vi "动力和环境监控系统首页.vi"() -> ()   [LabVIEW 2016, in "环境动力监测库.lvlib"]
uses:
  <vilib>/Utility/miscctls.llb/LVRowAndColumnTypeDef.ctl
  <vilib>/Utility/config.llb/NI_LVConfig.lvlib
  <vilib>/ptbypt/NI_PtbyPt.lvlib
panel:
  out "网络状态":bool
  in  "监测设备更新":bool
  in  "设备列表":i32(listbox)
  in  "add":bool
  out "设备当前时间:":timestamp format="%<%Y/%m/%d %H:%M:%S>T"
  out "当前传感器数量:":i32
  in  "设备":T1(ring)
  # "系统当前状态"
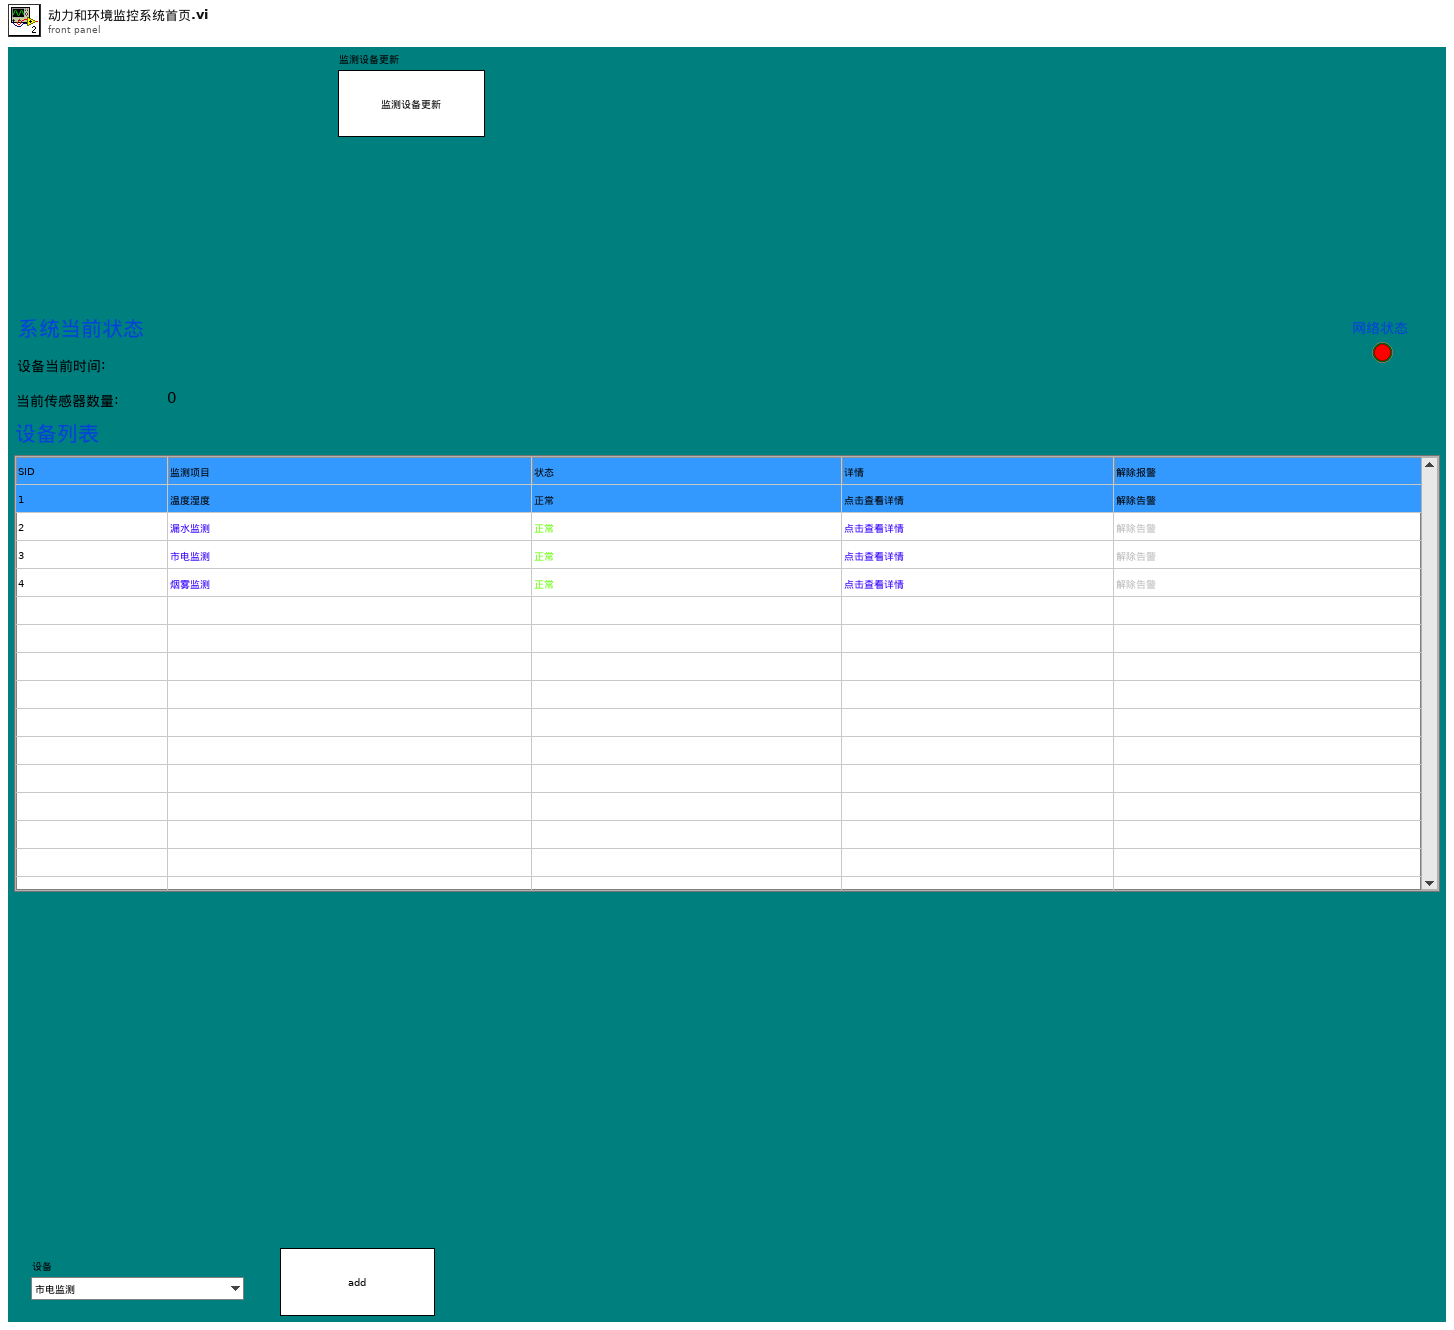
[diagram p1: front panel]
types:
  T1 = enum16{"市电监测", "UPS监测", "用水量监测", "空调监测", "烟雾监测", "温度湿度", "振动监测", "红外入侵监测", "漏水监测", "门禁开关监测", "视频监测"}
  T2 = typedef "NI_LVConfig.lvlib/Config Data RefNum.ctl" = refnum<k1>
  T3 = cluster{"市电监测":bool, "用水量监测":bool, "烟雾监测":bool, "温度湿度":bool, "振动监测":bool, "红外入侵监测":bool, "漏水监测":bool, "门禁开关监测":bool, "视频监测":bool, "UPS监测":bool, "空调监测":bool, "冰箱监测":bool, "排气扇监测":bool, "蓄电池监测":bool}
  T4 = enum32{"Invalid", "Standard", "Closed", "Hidden", "Minimized", "Maximized"}
  T5 = cluster{"漏水监测输出":bool, "门禁监测输出":bool, "温湿度监测输出":bool, "烟雾监测输出":bool, "空调监测输出":bool, "自动重合闸输出":bool, "红外入侵输出":bool, "振动输出":bool}
  T6 = typedef "LVRowAndColumnTypeDef.ctl" = cluster{"Row":i32, "Column":i32}
  T7 = typedef "LVPoint32TypeDef.ctl" = cluster{"Horizontal":i32, "Vertical":i32}
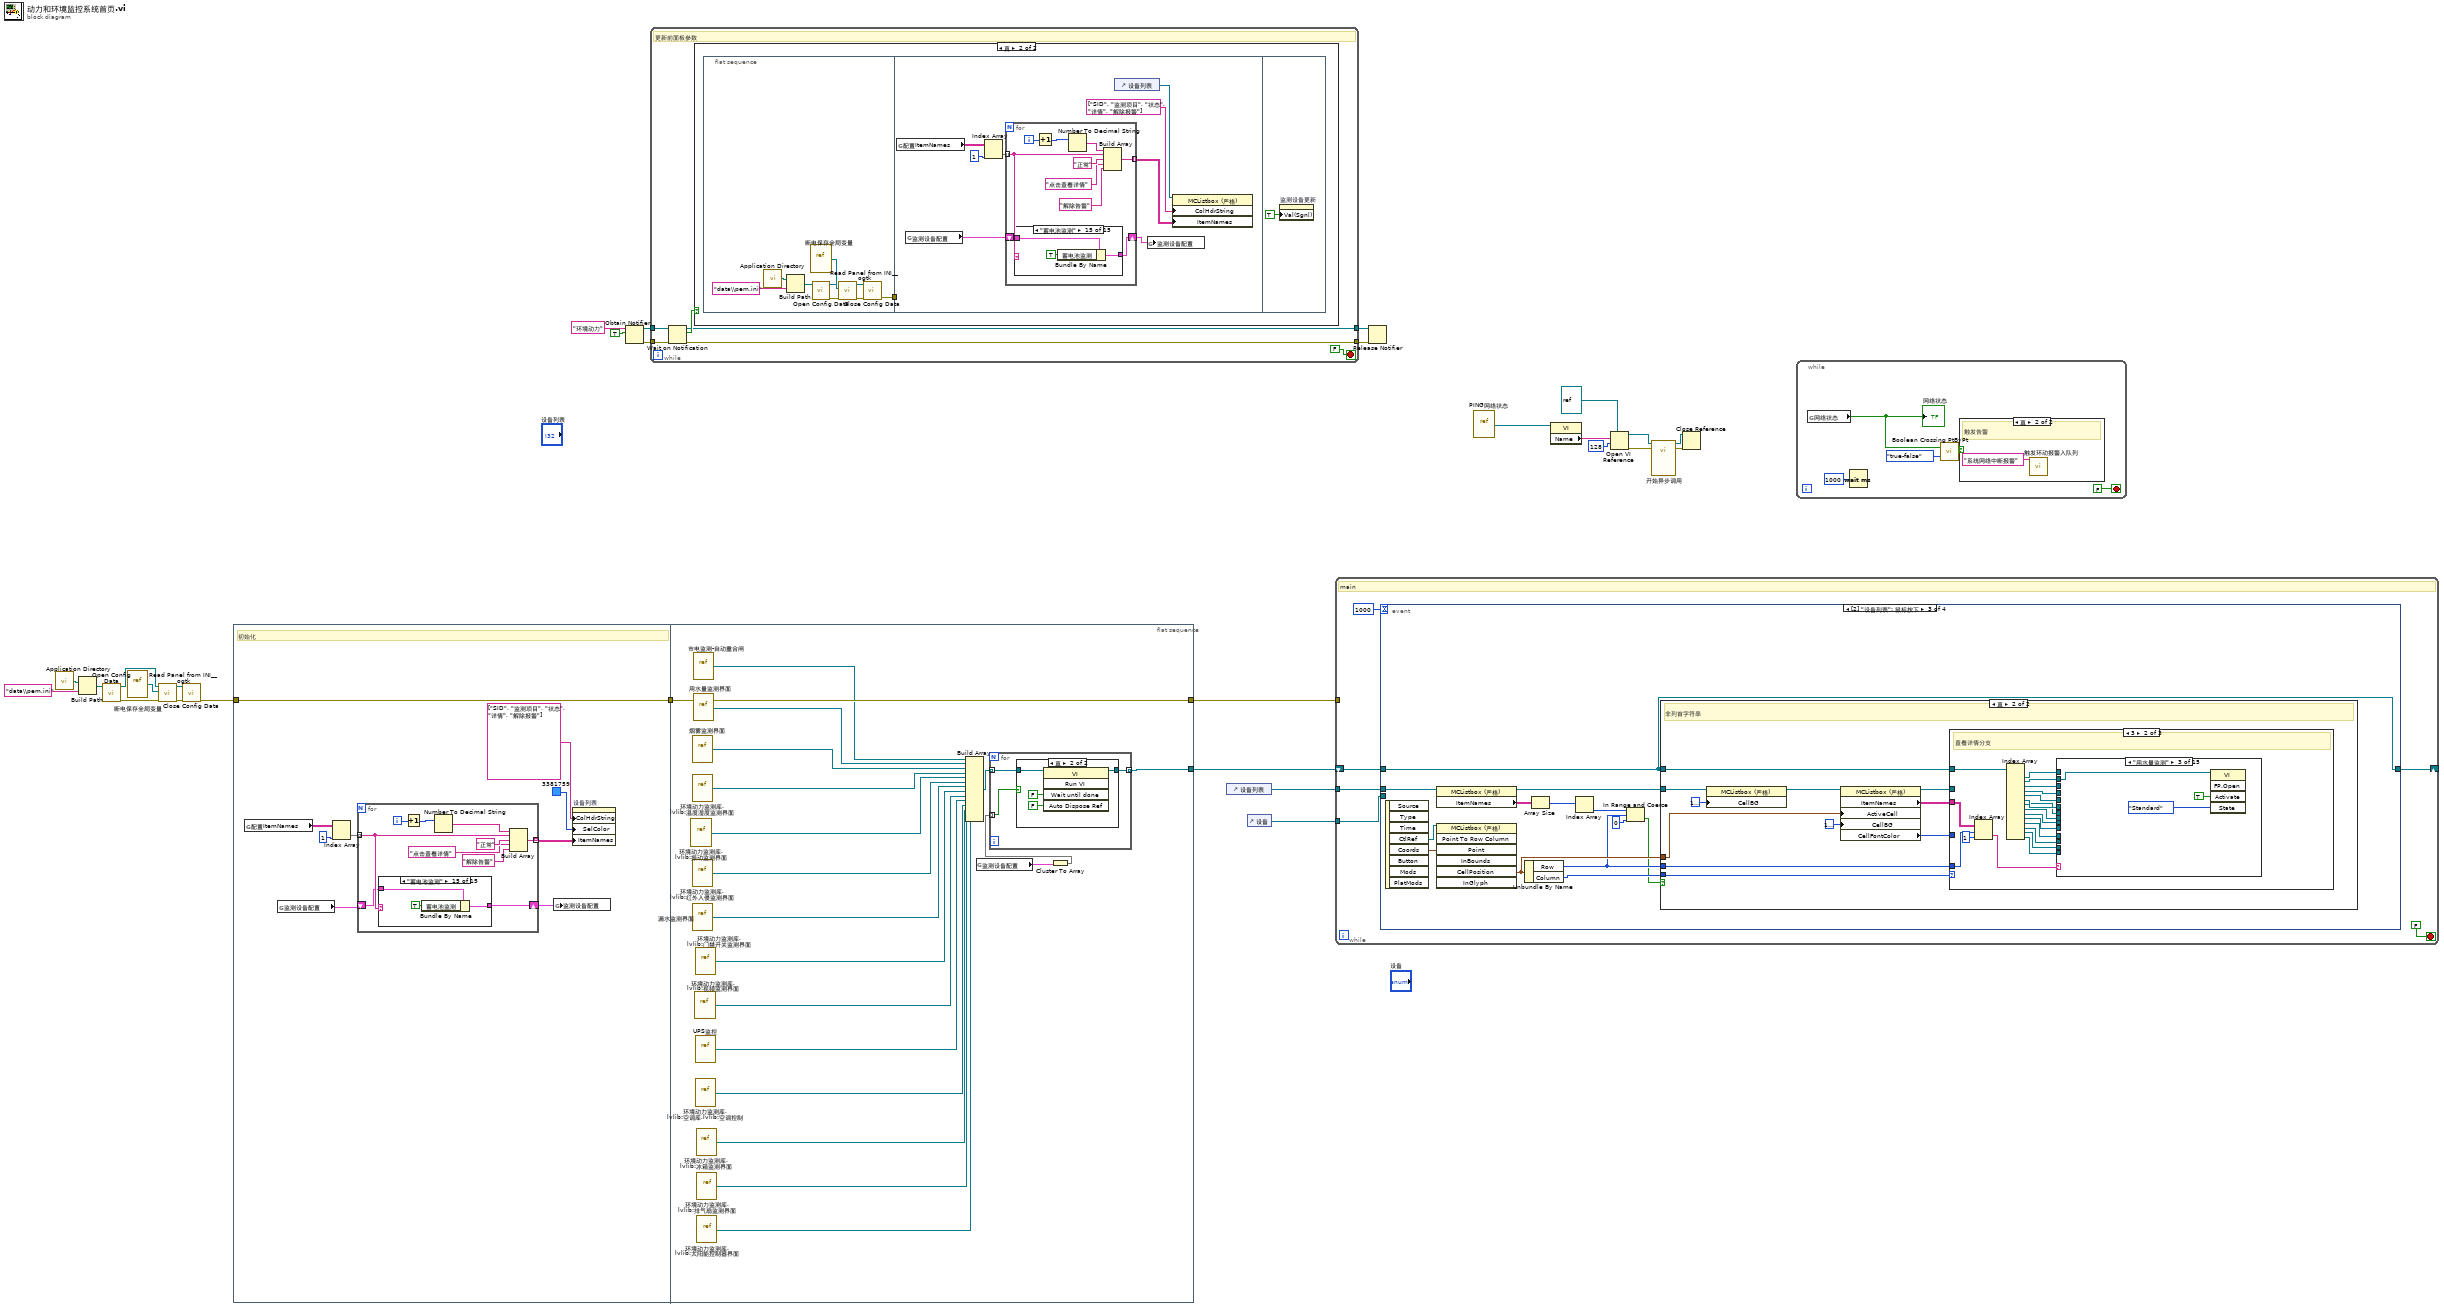
[diagram p0: block diagram]
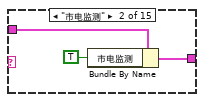
[diagram p5: hidden frame]
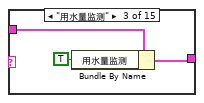
[diagram p6: hidden frame]
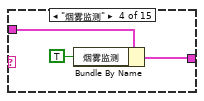
[diagram p7: hidden frame]
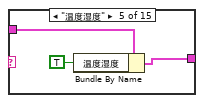
[diagram p8: hidden frame]
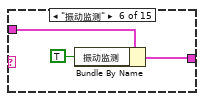
[diagram p9: hidden frame]
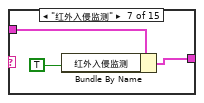
[diagram p10: hidden frame]
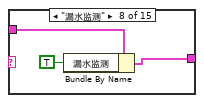
[diagram p11: hidden frame]
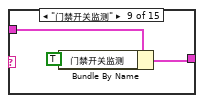
[diagram p12: hidden frame]
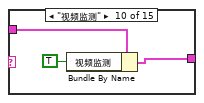
[diagram p13: hidden frame]
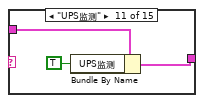
[diagram p14: hidden frame]
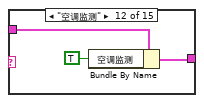
[diagram p15: hidden frame]
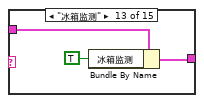
[diagram p16: hidden frame]
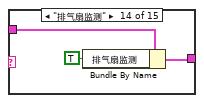
[diagram p17: hidden frame]
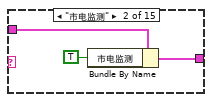
[diagram p19: hidden frame]
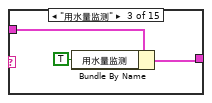
[diagram p20: hidden frame]
diagram:
  n1 = call <vilib>:"Application Directory.vi"() -> ("Application Directory"=w26:path)
  n2 = Build Path(base path=w26, name or relative path="data\\pem.ini" ("名称或相对路径")) -> (appended path=w24:path)
  n3 = call <vilib>:"Open Config Data.vi"("configuration file path"=w24) -> ("error out"=w20:errorcluster, "refnum"=w23:T2)  [unwired: 8 in, 1 out]
  n4 = vi-ref "断电保存全局变量.vi"() -> (w22:refnum<vi>)
  n5 = call <userlib>:"Read Panel from INI__ogtk.vi"("error in (no error)"=w20, "VI ref"=w22, "refnum"=w23) -> ("error out"=w19:errorcluster, "refnum out"=w21:T2)  [unwired: 7 in]
  n6 = call <vilib>:"Close Config Data.vi"("error in (no error)"=w19, "refnum"=w21) -> ("error out"=w18:errorcluster)  [unwired: 8 in, 1 out]
  n7 = flat-sequence {
    tunnel: w18 -> [w31]
    tunnel: [w31] -> w11
    tunnel: [w109] -> w9
    tunnel: w11 -> [w109]
    tunnel: [w95] -> w10
    frame #0 {
      # "初始化"
      n8 = global read "断电保存全局变量.vi" "配置ItemNames"() -> (w35:string[][])
      n9 = global read "断电保存全局变量.vi" "监测设备配置"() -> (w30:T3)
      n10 = Index Array(array=w35, index (col)=1 ("禁用的索引 (列)")) -> (element=w33:string[])  [unwired: 1 in]
      n11 = for {
        tunnel: w33 -> [w40] mode=indexing
        tunnel: [w41] -> w32 mode=indexing
        shift-right: [w38] -> w29
        shift-left: w30 -> [w39]
        i -> [w47]
        n12 = case shown="\"蓄电池监测\"" w40 {
          tunnel: w39 -> [w48 w51 w53 w56 w59 w62 w65 w68 w71 w74 w77 w80 w83 w86 w89]
          tunnel: [w48 w49 w52 w55 w58 w61 w64 w67 w70 w73 w76 w79 w82 w85 w88] -> w38
          frame "假", Default {
          }
          frame "市电监测" {
            n13 = Bundle By Name(cluster=w51, "市电监测"=TRUE) -> (w49:T3)
          }
          frame "用水量监测" {
            n14 = Bundle By Name(cluster=w53, "用水量监测"=TRUE ("市电监测")) -> (w52:T3)
          }
          frame "烟雾监测" {
            n15 = Bundle By Name(cluster=w56, "烟雾监测"=TRUE ("市电监测")) -> (w55:T3)
          }
          frame "温度湿度" {
            n16 = Bundle By Name(cluster=w59, "温度湿度"=TRUE ("市电监测")) -> (w58:T3)
          }
          frame "振动监测" {
            n17 = Bundle By Name(cluster=w62, "振动监测"=TRUE ("市电监测")) -> (w61:T3)
          }
          frame "红外入侵监测" {
            n18 = Bundle By Name(cluster=w65, "红外入侵监测"=TRUE ("市电监测")) -> (w64:T3)
          }
          frame "漏水监测" {
            n19 = Bundle By Name(cluster=w68, "漏水监测"=TRUE ("市电监测")) -> (w67:T3)
          }
          frame "门禁开关监测" {
            n20 = Bundle By Name(cluster=w71, "门禁开关监测"=TRUE ("市电监测")) -> (w70:T3)
          }
          frame "视频监测" {
            n21 = Bundle By Name(cluster=w74, "视频监测"=TRUE ("市电监测")) -> (w73:T3)
          }
          frame "UPS监测" {
            n22 = Bundle By Name(cluster=w77, "UPS监测"=TRUE ("市电监测")) -> (w76:T3)
          }
          frame "空调监测" {
            n23 = Bundle By Name(cluster=w80, "空调监测"=TRUE ("市电监测")) -> (w79:T3)
          }
          frame "冰箱监测" {
            n24 = Bundle By Name(cluster=w83, "冰箱监测"=TRUE ("市电监测")) -> (w82:T3)
          }
          frame "排气扇监测" {
            n25 = Bundle By Name(cluster=w86, "排气扇监测"=TRUE ("市电监测")) -> (w85:T3)
          }
          frame "蓄电池监测" {
            n26 = Bundle By Name(cluster=w89, "蓄电池监测"=TRUE ("市电监测")) -> (w88:T3)
          }
        }
        n27 = Increment(x=w47) -> (x+1=w46:i32)
        n28 = Number To Decimal String(number=w46) -> (decimal integer string=w45:string)  [unwired: 1 in]
        n29 = Build Array(w45, w40, "正常" ("元素"), "点击查看详情" ("元素"), "解除告警" ("元素")) -> (w41:string[])
      }
      n30 = global write "断电保存全局变量.vi" "监测设备配置"(w29) -> ()
      n31 = property on="设备列表" class="MCListbox (严格)"("ColHdrString"=string[] ["SID", "监测项目", "状态", "详情", "解除报警"] ("列首字符串[]"), "SelColor"=u32 3381759, "ItemNames"=w32) -> ()  [unwired: 2 in, 2 out]
    }
    frame #1 {
      n32 = vi-ref "环境动力监测库.lvlib:振动监测界面.vi"() -> (w101:refnum<vi>)
      n33 = vi-ref "烟雾监测界面.vi"() -> (w99:refnum<vi>)
      n34 = vi-ref "环境动力监测库.lvlib:温度湿度监测界面.vi"() -> (w100:refnum<vi>)
      n35 = vi-ref "环境动力监测库.lvlib:红外入侵监测界面.vi"() -> (w102:refnum<vi>)
      n36 = vi-ref "漏水监测界面.vi"() -> (w103:refnum<vi>)
      n37 = vi-ref "市电监测-自动重合闸.vi"() -> (w97:refnum<vi>)
      n38 = vi-ref "用水量监测界面.vi"() -> (w98:refnum<vi>)
      n39 = vi-ref "环境动力监测库.lvlib:视频监测界面.vi"() -> (w105:refnum<vi>)
      n40 = vi-ref "环境动力监测库.lvlib:门禁开关监测界面.vi"() -> (w104:refnum<vi>)
      n41 = vi-ref "UPS监控.vi"() -> (w106:refnum<vi>)
      n42 = vi-ref "环境动力监测库.lvlib:空调库.lvlib:空调控制.vi"() -> (w107:refnum<vi>)
      n43 = vi-ref "环境动力监测库.lvlib:冰箱监测界面.vi"() -> (w92:refnum<vi>)
      n44 = vi-ref "环境动力监测库.lvlib:排气扇监测界面.vi"() -> (w93:refnum<vi>)
      n45 = vi-ref "环境动力监测库.lvlib:太阳能控制器界面.vi"() -> (w94:refnum<vi>)
      n46 = Build Array(w97, w98, w99, w100, w101, w102, w103, w104, w105, w106, w107, w92, w93, w94) -> (w96:refnum<vi>[])
      n47 = global read "断电保存全局变量.vi" "监测设备配置"() -> (w91:T3)
      n48 = Cluster To Array(cluster=w91) -> (array=w108:bool[])
      n49 = for {
        tunnel: w96 -> [w112] mode=indexing
        tunnel: [w111] -> w95 mode=indexing
        tunnel: w108 -> [w110] mode=indexing
        n50 = case shown="真" w110 {
          tunnel: w112 -> [w113 w115]
          tunnel: [w113 w114] -> w111
          frame False {
          }
          frame True {
            n51 = invoke class="VI" method="Run VI"(reference=w115, "Wait until done"=FALSE ("结束前等待"), "Auto Dispose Ref"=FALSE ("自动销毁引用")) -> (reference out=w114:refnum<vi>)  [unwired: 2 in, 4 out]
          }
        }
      }
    }
  }
  n52 = Obtain Notifier(name (unnamed)="环境动力" ("名称（未命名）"), notification data type=TRUE) -> (notifier out=w17:refnum<notifier>, error out=w16:errorcluster)  [unwired: 2 in, 1 out]
  n53 = while {
    tunnel: w17 -> [w123]
    tunnel: w16 -> [w122]
    tunnel: [w119] -> w13
    tunnel: [w118] -> w12
    stop <- FALSE stop-if-true
    # "更新前面板参数"
    n54 = Wait on Notification(notifier=w123, error in (no error)=w122) -> (notifier out=w119:refnum<notifier>, notification=w121:bool, error out=w118:errorcluster)  [unwired: 2 in, 1 out]
    n55 = case shown="真" w121 {
      frame False {
      }
      frame True {
        n56 = flat-sequence {
          tunnel: [w125] -> w124
          tunnel: w124 -> [_]
          frame #0 {
            n57 = call <vilib>:"Application Directory.vi"() -> ("Application Directory"=w126:path)
            n58 = Build Path(base path=w126, name or relative path="data\\pem.ini" ("名称或相对路径")) -> (appended path=w128:path)
            n59 = vi-ref "断电保存全局变量.vi"() -> (w130:refnum<vi>)
            n60 = call <vilib>:"Open Config Data.vi"("configuration file path"=w128) -> ("error out"=w132:errorcluster, "refnum"=w129:T2)  [unwired: 8 in, 1 out]
            n61 = call <userlib>:"Read Panel from INI__ogtk.vi"("error in (no error)"=w132, "VI ref"=w130, "refnum"=w129) -> ("error out"=w133:errorcluster, "refnum out"=w131:T2)  [unwired: 7 in]
            n62 = call <vilib>:"Close Config Data.vi"("error in (no error)"=w133, "refnum"=w131) -> ("error out"=w125:errorcluster)  [unwired: 8 in, 1 out]
          }
          frame #1 {
            n63 = global read "断电保存全局变量.vi" "配置ItemNames"() -> (w136:string[][])
            n64 = global read "断电保存全局变量.vi" "监测设备配置"() -> (w135:T3)
            n65 = Index Array(array=w136, index (col)=1 ("禁用的索引 (列)")) -> (element=w138:string[])  [unwired: 1 in]
            n66 = for {
              tunnel: w138 -> [w142] mode=indexing
              tunnel: [w145] -> w141 mode=indexing
              shift-right: [w143] -> w134
              shift-left: w135 -> [w144]
              i -> [w151]
              n67 = case shown="\"蓄电池监测\"" w142 {
                tunnel: w144 -> [w152 w155 w157 w160 w163 w166 w169 w172 w175 w178 w181 w184 w187 w190 w193]
                tunnel: [w152 w153 w156 w159 w162 w165 w168 w171 w174 w177 w180 w183 w186 w189 w192] -> w143
                frame "假", Default {
                }
                frame "市电监测" {
                  n68 = Bundle By Name(cluster=w155, "市电监测"=TRUE) -> (w153:T3)
                }
                frame "用水量监测" {
                  n69 = Bundle By Name(cluster=w157, "用水量监测"=TRUE ("市电监测")) -> (w156:T3)
                }
                frame "烟雾监测" {
                  n70 = Bundle By Name(cluster=w160, "烟雾监测"=TRUE ("市电监测")) -> (w159:T3)
                }
                frame "温度湿度" {
                  n71 = Bundle By Name(cluster=w163, "温度湿度"=TRUE ("市电监测")) -> (w162:T3)
                }
                frame "振动监测" {
                  n72 = Bundle By Name(cluster=w166, "振动监测"=TRUE ("市电监测")) -> (w165:T3)
                }
                frame "红外入侵监测" {
                  n73 = Bundle By Name(cluster=w169, "红外入侵监测"=TRUE ("市电监测")) -> (w168:T3)
                }
                frame "漏水监测" {
                  n74 = Bundle By Name(cluster=w172, "漏水监测"=TRUE ("市电监测")) -> (w171:T3)
                }
                frame "门禁开关监测" {
                  n75 = Bundle By Name(cluster=w175, "门禁开关监测"=TRUE ("市电监测")) -> (w174:T3)
                }
                frame "视频监测" {
                  n76 = Bundle By Name(cluster=w178, "视频监测"=TRUE ("市电监测")) -> (w177:T3)
                }
                frame "UPS监测" {
                  n77 = Bundle By Name(cluster=w181, "UPS监测"=TRUE ("市电监测")) -> (w180:T3)
                }
                frame "空调监测" {
                  n78 = Bundle By Name(cluster=w184, "空调监测"=TRUE ("市电监测")) -> (w183:T3)
                }
                frame "冰箱监测" {
                  n79 = Bundle By Name(cluster=w187, "冰箱监测"=TRUE ("市电监测")) -> (w186:T3)
                }
                frame "排气扇监测" {
                  n80 = Bundle By Name(cluster=w190, "排气扇监测"=TRUE ("市电监测")) -> (w189:T3)
                }
                frame "蓄电池监测" {
                  n81 = Bundle By Name(cluster=w193, "蓄电池监测"=TRUE ("市电监测")) -> (w192:T3)
                }
              }
              n82 = Increment(x=w151) -> (x+1=w150:i32)
              n83 = Number To Decimal String(number=w150) -> (decimal integer string=w149:string)  [unwired: 1 in]
              n84 = Build Array(w149, w142, "正常" ("元素"), "点击查看详情" ("元素"), "解除告警" ("元素")) -> (w145:string[])
            }
            n85 = control-ref of="设备列表"() -> (w139:refnum<vi>)
            n86 = global write "断电保存全局变量.vi" "监测设备配置"(w134) -> ()
            n87 = property class="MCListbox (严格)"(reference=w139, "ColHdrString"=string[] ["SID", "监测项目", "状态", "详情", "解除报警"] ("列首字符串[]"), "ItemNames"=w141) -> ()  [unwired: 1 in, 2 out]
          }
          frame #2 {
            n88 = property on="监测设备更新" class="Bool (严格)"("Val(Sgnl)"=TRUE ("值(信号)")) -> ()  [unwired: 2 in, 2 out]
          }
        }
      }
    }
  }
  n89 = control-ref of="设备列表"() -> (w28:refnum<vi>)
  n90 = control-ref of="设备"() -> (w27:refnum<vi>)
  n91 = while {
    tunnel: w28 -> [w200]
    tunnel: w27 -> [w199]
    tunnel: w9 -> [_]
    shift-right: [w196] -> _
    shift-left: w10 -> [w197]
    stop <- FALSE stop-if-true
    # "main"
    n92 = event shown="[2] \"设备列表\": 鼠标按下" {
      selector: _ -> [_ _ _ _]
      dyn-events: _ -> [_ _ _ _]
      timeout: 1000 -> [_ _ _ _]
      tunnel: w200 -> [_ w284 w291 _]
      tunnel: w199 -> [_ w283 _ _]
      tunnel: w197 -> [w203 w258 w285 w388]
      tunnel: [w203 w258 w285 w387] -> w196
      event Timeout {
        n93 = event-data() -> ()  [unwired: 1 in, 3 out]
        n94 = Get Date/Time In Seconds() -> (seconds since 1Jan1904=→"设备当前时间:":timestamp)
        n95 = property on="设备列表" class="MCListbox (严格)"() -> (error out=w205:errorcluster, "ItemNames"=w214:string[][])  [unwired: 2 in, 1 out]
        n96 = global read "断电保存全局变量.vi" "监测配置输出"() -> (w202:T5)
        n97 = Array Size(array=w214) -> (size(s)=w220:i32[])
        n98 = Index Array(array=w214, index (col) #1=1 ("禁用的索引 (列)"), index (col) #2=2 ("索引 (列)")) -> (element #1=w212:string[], element #2=w210:string[])  [unwired: 2 in]
        n99 = Index Array(array=w220) -> (element=w215:i32)  [unwired: 1 in]
        "当前传感器数量:" <- w215
        n100 = for {
          tunnel: w212 -> [w236] mode=indexing
          tunnel: w202 -> [w235]
          shift-right: [w231] -> w207
          shift-left: w210 -> [w233]
          tunnel: w205 -> [w227]
          tunnel: [w226] -> w204
          i -> [w224]
          w225 = T6 {"Row"=0, "Column"=0} ("活动单元格:活动单元格")
          n101 = case shown="\"烟雾监测\"" w236 {
            tunnel: w235 -> [_ w245 w247 w249 w251 w253 w255]
            tunnel: [TRUE ("烟雾监测输出") w244 w246 w248 w250 w252 w254] -> w234
            frame "假", Default {
            }
            frame "市电监测" {
              n102 = Unbundle By Name(w245) -> ("自动重合闸输出"=w244:bool)
            }
            frame "空调监测" {
              n103 = Unbundle By Name(w247) -> ("空调监测输出"=w246:bool)
            }
            frame "漏水监测" {
              n104 = Unbundle By Name(w249) -> ("漏水监测输出"=w248:bool)
            }
            frame "门禁开关监测" {
              n105 = Unbundle By Name(w251) -> ("门禁监测输出"=w250:bool)
            }
            frame "温度湿度" {
              n106 = Unbundle By Name(w253) -> ("温湿度监测输出"=w252:bool)
            }
            frame "烟雾监测" {
              n107 = Unbundle By Name(w255) -> ("烟雾监测输出"=w254:bool)
            }
          }
          n108 = case shown="假" w234 {
            tunnel: ["报警" "正常"] -> w232
            tunnel: [u32 16711680 u32 6618880] -> w228
            tunnel: [u32 3342591 ("颜色盒") u32 12369084] -> w221
            frame False {
            }
            frame True {
            }
          }
          n109 = Bundle By Name(cluster=w225, "Row"=w224, "Column"=2) -> (w229:T6)
          n110 = Bundle By Name(cluster=w225, "Row"=w224, "Column"=4) -> (w222:T6)
          n111 = property on="设备列表" class="MCListbox (严格)"(error in=w227, "ActiveCell"=w229, "CellFontColor"=w228, "ActiveCell"=w222, "CellFontColor"=w221) -> (error out=w226:errorcluster)  [unwired: 1 in, 1 out]
          n112 = Replace Array Subset(array=w233, new element=w232, index=w224) -> (w231:string[])
        }
        n113 = for {
          N: w215 -> [_]
          tunnel: [w256] -> w219 mode=indexing
          i -> [w257]
          n114 = Increment(x=w257) -> (x+1=w256:i32)
        }
        n115 = Number To Decimal String(number=w219) -> (decimal integer string=w218:string[])  [unwired: 1 in]
        n116 = Replace Array Subset(array=w214, new element=w218, index (col)=0 ("禁用的索引 (列)")) -> (w209:string[][])  [unwired: 1 in]
        n117 = Replace Array Subset(array=w209, new element=w207, index (col)=2 ("禁用的索引 (列)")) -> (w206:string[][])  [unwired: 1 in]
        n118 = property on="设备列表" class="MCListbox (严格)"(error in=w204, "ItemNames"=w206) -> ()  [unwired: 1 in, 2 out]
      }
      event "add": Value Change {
        w260 = u32 3342591 ("颜色盒")
        n119 = event-data() -> ()  [unwired: 1 in, 6 out]
        n120 = property class="MCListbox (严格)"(reference=w284) -> (reference out=w273:refnum<vi>, "ItemNames"=w277:string[][])  [unwired: 1 in, 1 out]
        n121 = property class="Enum (严格)"(reference=w283) -> ("RingText.Text"=w282:string)  [unwired: 1 in, 2 out]
        n122 = Array Size(array=w277) -> (size(s)=w276:i32[])
        n123 = Index Array(array=w276) -> (element=w265:i32)  [unwired: 1 in]
        n124 = Increment(x=w265) -> (x+1=w275:i32)
        n125 = Number To Decimal String(number=w275) -> (decimal integer string=w274:string)  [unwired: 1 in]
        n126 = Build Array(w274, w282, "正常" ("元素"), "点击查看详情" ("元素"), "解除告警" ("元素")) -> (w281:string[])
        n127 = Build Array (concatenate)(w277, w281) -> (w262:string[][])
        n128 = Bundle(w265, "Column"=1) -> (w261:cluster{i32, "Column":i32})  [unwired: 1 in]
        n129 = Bundle(w265, "Column"=2) -> (w270:cluster{i32, "Column":i32})  [unwired: 1 in]
        n130 = Bundle(w265, "Column"=3) -> (w267:cluster{i32, "Column":i32})  [unwired: 1 in]
        n131 = Bundle(w265, "Column"=4) -> (w264:cluster{i32, "Column":i32})  [unwired: 1 in]
        n132 = property class="MCListbox (严格)"(reference=w273, "ItemNames"=w262, "ActiveCell"=w261, "CellFontColor"=w260, "CellFontBold"=TRUE ("活动单元格:单元格字体:斜体"), "ActiveCell"=w270, "CellFontColor"=u32 61277 ("颜色盒"), "ActiveCell"=w267, "CellFontColor"=w260, "ActiveCell"=w264, "CellFontColor"=u32 12369084 ("颜色盒")) -> ()  [unwired: 1 in, 2 out]
      }
      event "设备列表": Mouse Down {
        n133 = event-data() -> ("CtlRef"=w297:refnum<vi>, "Coords"=w295:T7)  [unwired: 1 in, 6 out]
        n134 = property class="MCListbox (严格)"(reference=w291) -> (reference out=w287:refnum<vi>, "ItemNames"=w290:string[][])  [unwired: 1 in, 1 out]
        n135 = invoke class="MCListbox (严格)" method="Point To Row Column"(reference=w297, "Point"=w295) -> ("CellPosition"=w294:T6)  [unwired: 5 in, 6 out]
        n136 = Unbundle By Name(w294) -> ("Row"=w293:i32, "Column"=w296:i32)
        n137 = Array Size(array=w290) -> (size(s)=w289:i32[])
        n138 = Index Array(array=w289) -> (element=w288:i32)  [unwired: 1 in]
        n139 = In Range and Coerce(upper limit=w288, x=w293, lower limit=0 ("下限")) -> (In Range?=w286:bool)  [unwired: 1 out]
        n140 = case shown="真" w286 {
          tunnel: w296 -> [_ w307]
          tunnel: w293 -> [_ w306]
          tunnel: w294 -> [_ w304]
          tunnel: w287 -> [_ w301]
          tunnel: w285 -> [_ w298]
          frame False {
          }
          frame True {
            # "非列首字符串"
            n141 = property class="MCListbox (严格)"(reference=w301, "CellBG"=u32 16777216) -> (reference out=w302:refnum<vi>)  [unwired: 1 in, 1 out]
            n142 = property class="MCListbox (严格)"(reference=w302, "ActiveCell"=w304, "CellBG"=u32 16777216) -> (reference out=w305:refnum<vi>, "ItemNames"=w308:string[][], "CellFontColor"=w299:u32)  [unwired: 1 in, 1 out]
            n143 = case shown="3" w307 {
              tunnel: w308 -> [_ w327 w378]
              tunnel: w306 -> [_ w325 w376]
              tunnel: w305 -> [_ _ w377]
              tunnel: w299 -> [_ _ w375]
              tunnel: w298 -> [_ w323 _]
              frame 0, Default {
              }
              frame 3 {
                # "查看详情分支"
                n144 = Index Array(array=w327, index (row)=w325, index (col)=1 ("禁用的索引 (列)")) -> (element=w324:string)
                n145 = Index Array(array=w323) -> (element #1=w322:refnum<vi>, element #2=w321:refnum<vi>, element #3=w320:refnum<vi>, element #4=w319:refnum<vi>, element #5=w318:refnum<vi>, element #6=w317:refnum<vi>, element #7=w316:refnum<vi>, element #8=w315:refnum<vi>, element #9=w314:refnum<vi>, element #10=w313:refnum<vi>, element #11=w312:refnum<vi>, element #12=w311:refnum<vi>, element #13=w309:refnum<vi>, element #14=w310:refnum<vi>)  [unwired: 14 in]
                n146 = case shown="\"用水量监测\"" w324 {
                  selector: w324 -> [w328 _ _ _ _ _ _ _ _ _ _ _ _ _ _]
                  tunnel: w322 -> [_ w331 _ _ _ _ _ _ _ _ _ _ _ _ _]
                  tunnel: w321 -> [_ _ w334 _ _ _ _ _ _ _ _ _ _ _ _]
                  tunnel: w320 -> [_ _ _ w337 _ _ _ _ _ _ _ _ _ _ _]
                  tunnel: w319 -> [_ _ _ _ w340 _ _ _ _ _ _ _ _ _ _]
                  tunnel: w318 -> [_ _ _ _ _ w343 _ _ _ _ _ _ _ _ _]
                  tunnel: w317 -> [_ _ _ _ _ _ w346 _ _ _ _ _ _ _ _]
                  tunnel: w316 -> [_ _ _ _ _ _ _ w349 _ _ _ _ _ _ _]
                  tunnel: w315 -> [_ _ _ _ _ _ _ _ w352 _ _ _ _ _ _]
                  tunnel: w314 -> [_ _ _ _ _ _ _ _ _ w355 _ _ _ _ _]
                  tunnel: w313 -> [_ _ _ _ _ _ _ _ _ _ w358 _ _ _ _]
                  tunnel: w312 -> [_ _ _ _ _ _ _ _ _ _ _ w361 _ _ _]
                  tunnel: w311 -> [_ _ _ _ _ _ _ _ _ _ _ _ w364 _ _]
                  tunnel: w310 -> [_ _ _ _ _ _ _ _ _ _ _ _ _ _ w370]
                  tunnel: w309 -> [_ _ _ _ _ _ _ _ _ _ _ _ _ w367 _]
                  frame "假", Default {
                    n147 = Concatenate Strings(w328, "详情" ("字符串")) -> (w330:string)
                    n148 = One Button Dialog(message=w330) -> ()  [unwired: 1 in, 1 out]
                  }
                  frame "市电监测" {
                    n149 = invoke class="VI" method="FP.Open"(reference=w331, "Activate"=TRUE ("激活？"), "State"=T4."Standard" ("状态")) -> ()  [unwired: 2 in, 5 out]
                  }
                  frame "用水量监测" {
                    n150 = invoke class="VI" method="FP.Open"(reference=w334, "Activate"=TRUE ("激活？"), "State"=T4."Standard" ("状态")) -> ()  [unwired: 2 in, 5 out]
                  }
                  frame "烟雾监测" {
                    n151 = invoke class="VI" method="FP.Open"(reference=w337, "Activate"=TRUE ("激活？"), "State"=T4."Standard" ("状态")) -> ()  [unwired: 2 in, 5 out]
                  }
                  frame "温度湿度" {
                    n152 = invoke class="VI" method="FP.Open"(reference=w340, "Activate"=TRUE ("激活？"), "State"=T4."Standard" ("状态")) -> ()  [unwired: 2 in, 5 out]
                  }
                  frame "振动监测" {
                    n153 = invoke class="VI" method="FP.Open"(reference=w343, "Activate"=TRUE ("激活？"), "State"=T4."Standard" ("状态")) -> ()  [unwired: 2 in, 5 out]
                  }
                  frame "红外入侵监测" {
                    n154 = invoke class="VI" method="FP.Open"(reference=w346, "Activate"=TRUE ("激活？"), "State"=T4."Standard" ("状态")) -> ()  [unwired: 2 in, 5 out]
                  }
                  frame "漏水监测" {
                    n155 = invoke class="VI" method="FP.Open"(reference=w349, "Activate"=TRUE ("激活？"), "State"=T4."Standard" ("状态")) -> ()  [unwired: 2 in, 5 out]
                  }
                  frame "门禁开关监测" {
                    n156 = invoke class="VI" method="FP.Open"(reference=w352, "Activate"=TRUE ("激活？"), "State"=T4."Standard" ("状态")) -> ()  [unwired: 2 in, 5 out]
                  }
                  frame "视频监测" {
                    n157 = invoke class="VI" method="FP.Open"(reference=w355, "Activate"=TRUE ("激活？"), "State"=T4."Standard" ("状态")) -> ()  [unwired: 2 in, 5 out]
                  }
                  frame "UPS监测" {
                    n158 = invoke class="VI" method="FP.Open"(reference=w358, "Activate"=TRUE ("激活？"), "State"=T4."Standard" ("状态")) -> ()  [unwired: 2 in, 5 out]
                  }
                  frame "空调监测" {
                    n159 = invoke class="VI" method="FP.Open"(reference=w361, "Activate"=TRUE ("激活？"), "State"=T4."Standard" ("状态")) -> ()  [unwired: 2 in, 5 out]
                  }
                  frame "冰箱监测" {
                    n160 = invoke class="VI" method="FP.Open"(reference=w364, "Activate"=TRUE ("激活？"), "State"=T4."Standard" ("状态")) -> ()  [unwired: 2 in, 5 out]
                  }
                  frame "排气扇监测" {
                    n161 = invoke class="VI" method="FP.Open"(reference=w367, "Activate"=TRUE ("激活？"), "State"=T4."Standard" ("状态")) -> ()  [unwired: 2 in, 5 out]
                  }
                  frame "蓄电池监测" {
                    n162 = invoke class="VI" method="FP.Open"(reference=w370, "Activate"=TRUE ("激活？"), "State"=T4."Standard" ("状态")) -> ()  [unwired: 2 in, 5 out]
                  }
                }
              }
              frame 4 {
                # "解除报警"
                n163 = Equal?(x=w375, y=u32 3342591 ("颜色盒")) -> (x = y?=w374:bool)
                n164 = case shown="真" w374 {
                  tunnel: w378 -> [_ w383]
                  tunnel: w377 -> [_ _]
                  tunnel: w376 -> [_ w382]
                  frame False {
                  }
                  frame True {
                    n165 = Index Array(array=w383, index (row)=w382, index (col)=1 ("禁用的索引 (列)")) -> (element=w380:string)
                    n166 = Format Into String(format string="是否解除%s报警？" ("消息"), w380) -> (resulting string=w384:string)  [unwired: 2 in, 1 out]
                    n167 = Two Button Dialog(message=w384) -> (T button?=w379:bool)  [unwired: 2 in]
                    n168 = case shown="真" w379 {
                      frame False {
                      }
                      frame True {
                        # "触发解除报警事件"
                      }
                    }
                  }
                }
              }
            }
          }
        }
      }
      event "监测设备更新": Value Change {
        n169 = event-data() -> ()  [unwired: 1 in, 6 out]
        n170 = global read "断电保存全局变量.vi" "监测设备配置"() -> (w386:T3)
        n171 = Cluster To Array(cluster=w386) -> (array=w389:bool[])
        n172 = for {
          tunnel: w388 -> [w392] mode=indexing
          tunnel: [w391] -> w387 mode=indexing
          tunnel: w389 -> [w390] mode=indexing
          n173 = case shown="真" w390 {
            tunnel: w392 -> [w393 w395]
            tunnel: [w393 w394] -> w391
            frame False {
            }
            frame True {
              n174 = invoke class="VI" method="Run VI"(reference=w395, "Wait until done"=FALSE ("结束前等待"), "Auto Dispose Ref"=FALSE ("自动销毁引用")) -> (reference out=w394:refnum<vi>)  [unwired: 2 in, 4 out]
            }
          }
        }
      }
    }
  }
  n175 = Release Notifier(notifier=w13, error in (no error)=w12) -> ()  [unwired: 1 in, 3 out]
  n176 = vi-ref "PING网络状态.vi"() -> (w1:refnum<vi>)
  n177 = property class="VI"(reference=w1) -> ("Name"=w8:string)  [unwired: 1 in, 2 out]
  n178 = Open VI Reference(type specifier VI Refnum (for type only)=refnum<vi> refnum, vi path=w8, options=128 ("选项")) -> (vi reference=w6:refnum<vi>, error out=w4:errorcluster)  [unwired: 3 in]
  n179 = call-by-ref "开始异步调用"(reference=w6, error in=w4) -> (reference out=w2:refnum<vi>, error out=w3:errorcluster)  [unwired: 12 in]
  n180 = Close Reference(reference=w2, error in (no error)=w3) -> ()  [unwired: 1 out]
  n181 = while {
    stop <- FALSE stop-if-true
    n182 = global read "内部交互全局变量.vi" "网络状态"() -> (w398:bool)
    "网络状态" <- w398
    n183 = Wait (ms)(milliseconds to wait=u32 1000 ("等待时间（毫秒）")) -> ()  [unwired: 1 out]
    n184 = call <vilib>:"Boolean Crossing PtByPt.vi"("direction"=enum16{"either", "false-true", "true-false"}."true-false", "input"=w398) -> ("crossing"=w399:bool)  [unwired: 1 in]
    n185 = case shown="真" w399 {
      frame False {
      }
      frame True {
        # "触发告警"
        n186 = call "触发环动报警入队列.vi"("报警内容"="系统网络中断报警") -> ()  [unwired: 11 in]
      }
    }
  }
